vi "Connection Handler VI.vi"(9 "Additional Data":variant, 10 "connection ID":T1, 11 "TCP Server Refnum":refnum<class "JKI TCP Server.lvclass">) -> ()   [LabVIEW 2020]
uses:
  <vilib>/addons/_JKI.lib/_JKI_lib_TCP_Server.llb/TCP Server Connection Session ID Cluster.ctl
  <vilib>/addons/_JKI.lib/_JKI_lib_TCP_Server.llb/JKI TCP Server.lvclass
  bd168d05-2ccd-4f69-90c9-be1b4e621865.vi
  316abe05-dd11-44a4-98b3-32ea1594dc48.vi
  a7f8194b-54d4-448d-8a65-d0b66a8fd47c.vi
  8a9da1d4-9237-4126-a3a1-8a9d876b672d.vi
  eb58fbab-51b7-4bfd-aab6-475a21a34b28.vi
  <userlib>/_NEVSTOP/Communicable State Machine(CSM)/_Support/Common/Trim Single line Text.vi
  <userlib>/_NEVSTOP/Communicable State Machine(CSM)/AdvanceAPI/CSM - Make String Arguments Safe.vi
  <userlib>/_NEVSTOP/Communicable State Machine(CSM)/AdvanceAPI/CSM - Keywords.vi
  <userlib>/_NEVSTOP/Communicable State Machine(CSM)/addons/API-String-Arugments-Support/_Support/Data To API String Arguments.vi
  _support/Module/CSM-TCP-Router.lvlib
  <userlib>/_NEVSTOP/Communicable State Machine(CSM)/Communicable State Machine.lvlib
  <userlib>/_NEVSTOP/Communicable State Machine(CSM)/_csmHelper/API with lvcsm Support/CSM-Helper API with lvcsm Support.lvlib
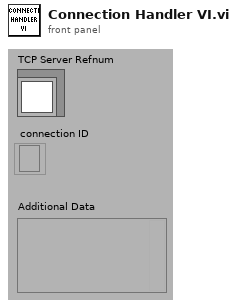
[diagram p1: front panel]
types:
  T1 = typedef "JKI TCP Server.lvclass/TCP Server Connection Session ID Cluster.ctl" = refnum<k5>
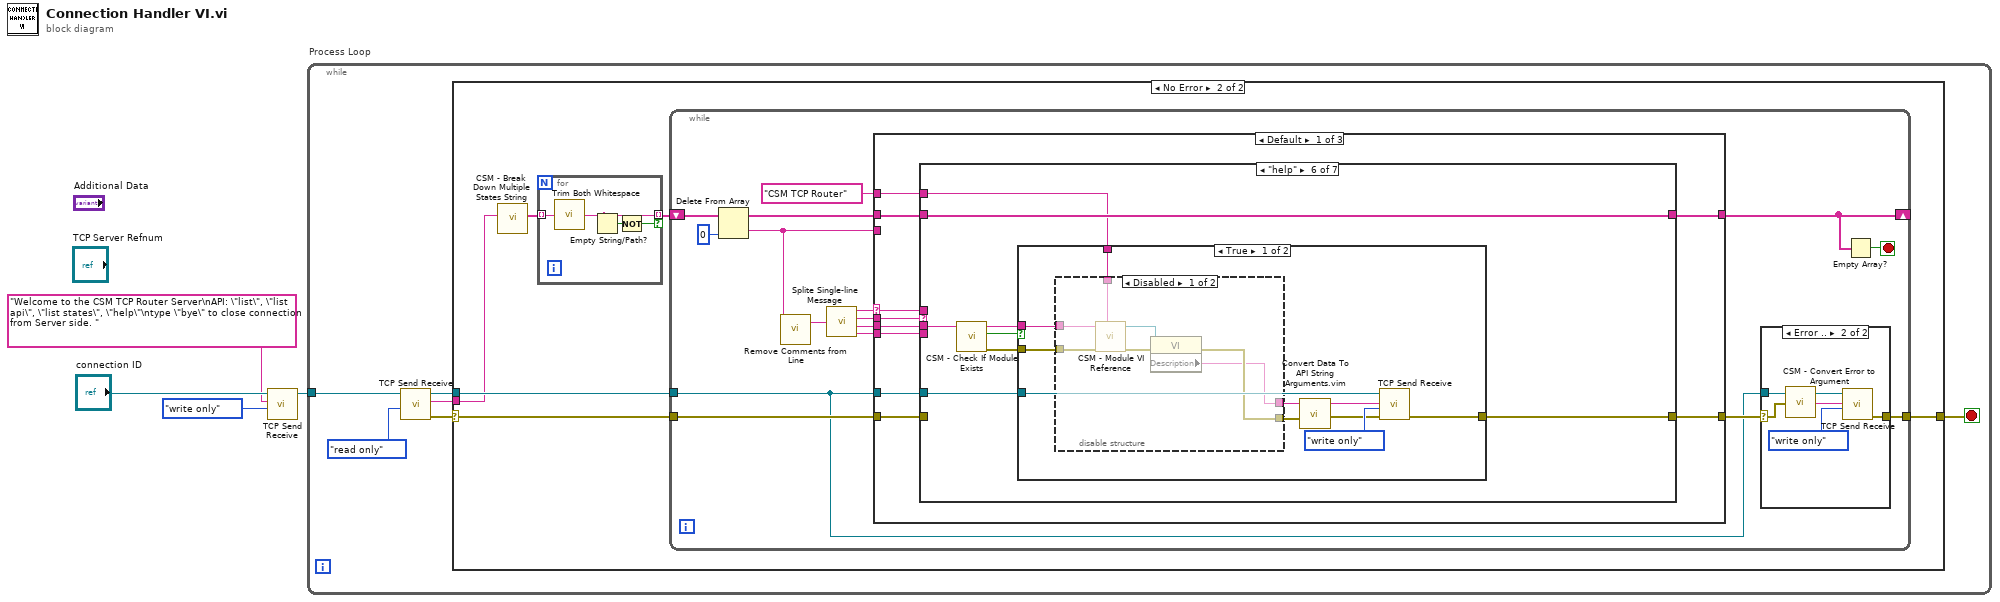
[diagram p0: block diagram]
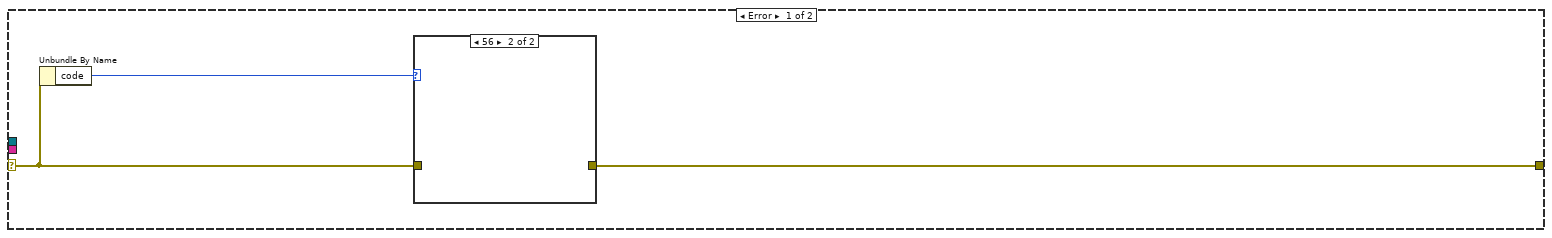
[diagram p2: hidden frame]
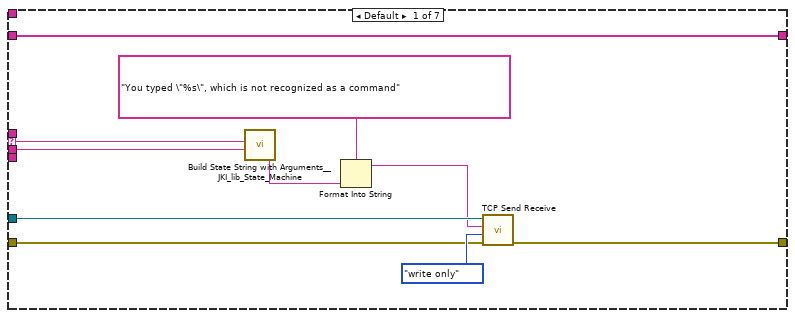
[diagram p5: hidden frame]
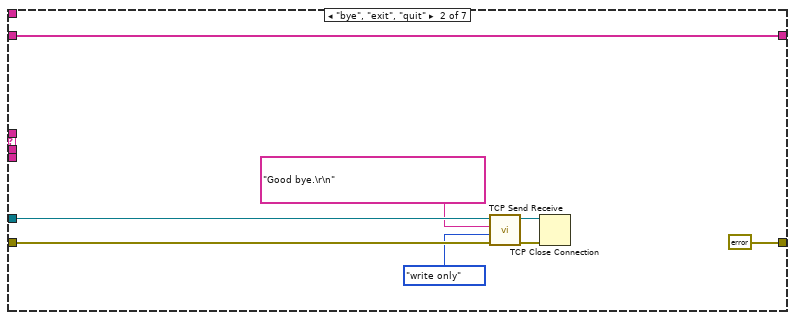
[diagram p6: hidden frame]
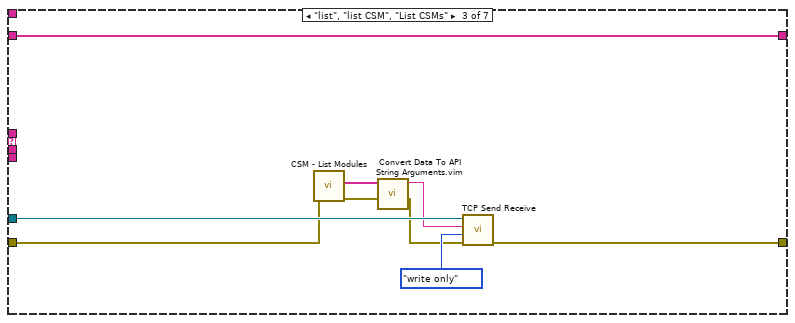
[diagram p7: hidden frame]
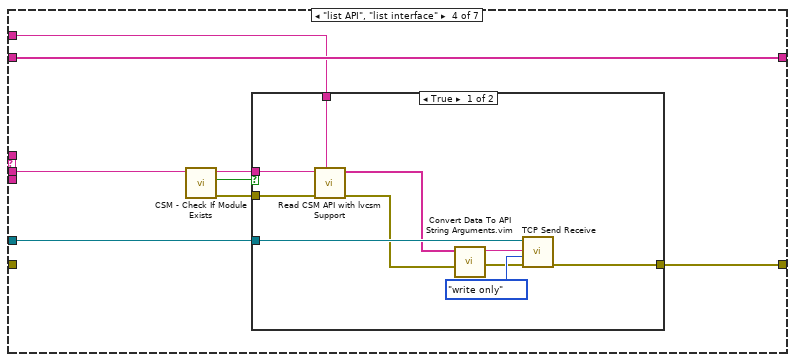
[diagram p8: hidden frame]
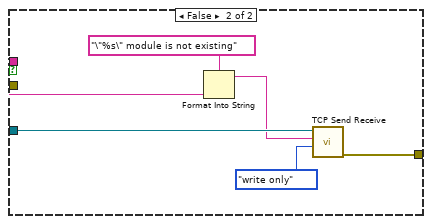
[diagram p9: hidden frame]
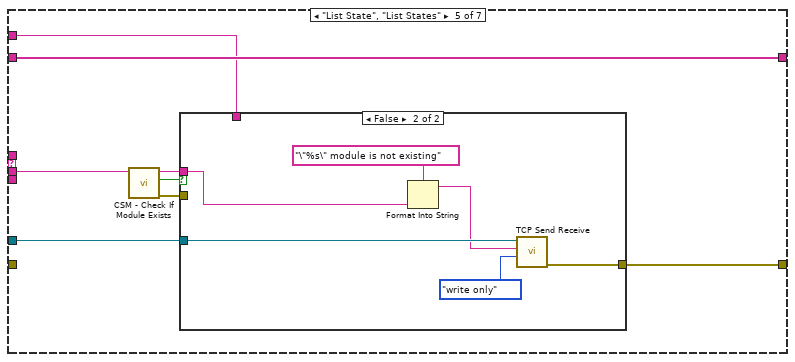
[diagram p10: hidden frame]
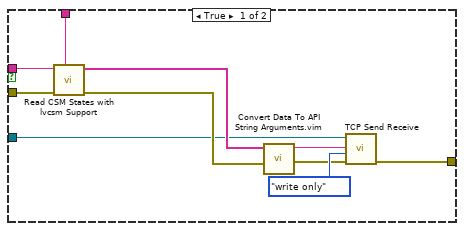
[diagram p11: hidden frame]
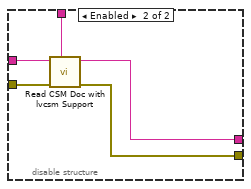
[diagram p12: hidden frame]
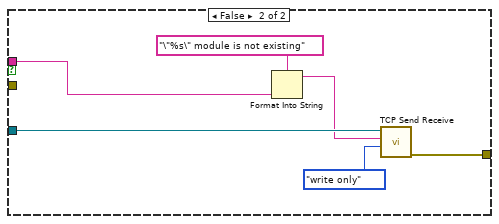
[diagram p13: hidden frame]
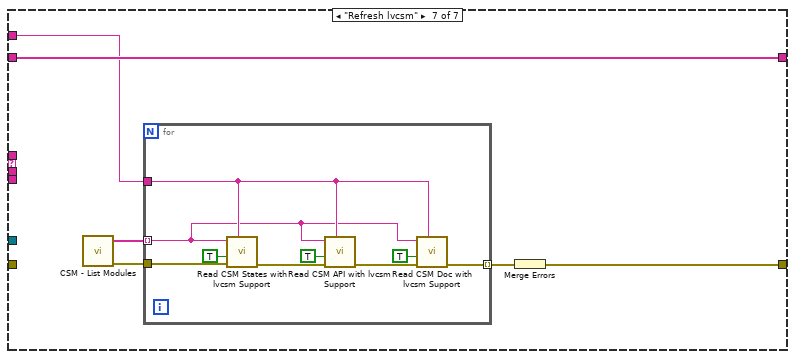
[diagram p14: hidden frame]
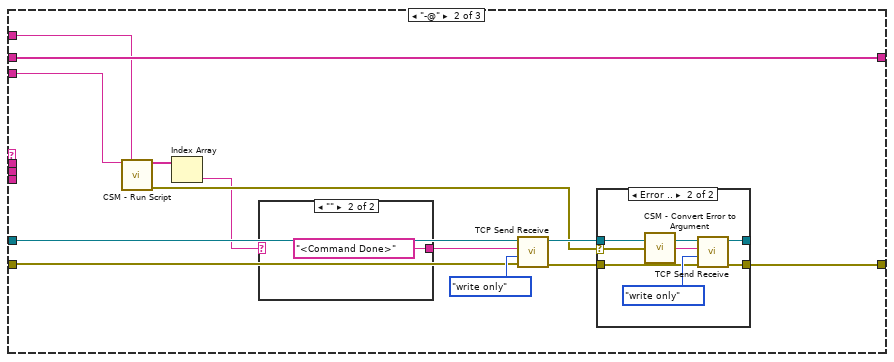
[diagram p15: hidden frame]
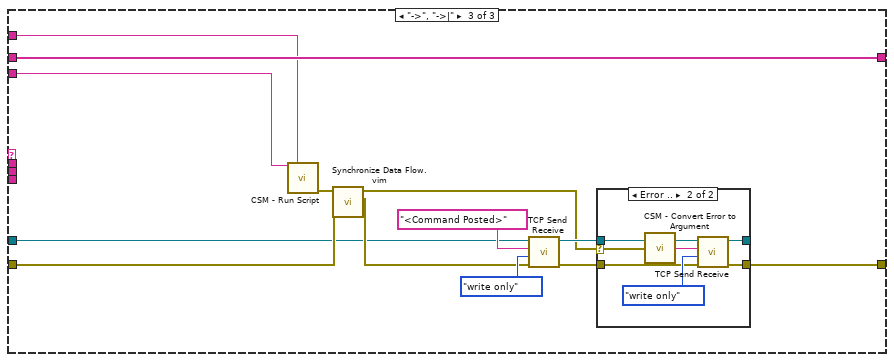
[diagram p18: hidden frame]
diagram:
  n1 = call "TCP Send Receive.vi"("access (read/write)"=enum16{"read/write", "read only", "write only"}."write only", "Data In"="Welcome to the CSM TCP Router Server\nAPI: \"list\", \"list api\", \"list states\", \"help\"\ntype \"bye\" to close connection from Server side. " ("data in"), "connection ID"="connection ID") -> ("connection ID Out"=w3:refnum<k5>)  [unwired: 6 in, 2 out]
  n2 = while "Process Loop" {
    tunnel: w3 -> [w9]
    stop <- w10 stop-if-true
    n3 = call "TCP Send Receive.vi"("access (read/write)"=enum16{"read/write", "read only", "write only"}."read only", "connection ID"=w9) -> ("error out"=w6:errorcluster, "Data Out"=w5:string, "connection ID Out"=w8:refnum<k5>)  [unwired: 7 in]
    n4 = case shown="No Error" w6 {
      selector: w6 -> [w12 w18]
      tunnel: w8 -> [_ w20]
      tunnel: w5 -> [_ w17]
      tunnel: [w11 w19] -> w10
      frame Error {
        n5 = Unbundle By Name(w12) -> ("code"=w13:i32)
        n6 = case shown="56" w13 {
          tunnel: w12 -> [w14 _]
          tunnel: [w14 _] -> w11
          frame 0, Default {
          }
          frame 56 {
          }
        }
      }
      frame No Error {
        n7 = call <userlib>:"CSM - Break Down Multiple States String.vi"("States"=w17) -> ("Multiple States"=w16:string[])  [unwired: 10 in]
        n8 = for {
          tunnel: w16 -> [w24] mode=indexing
          tunnel: [w23] -> w15 mode=indexing if=w21
          n9 = call <userlib>:"Trim Both Whitespace.vi"("string"=w24) -> ("trimmed string"=w23:string)  [unwired: 1 in]
          n10 = Empty String/Path?(string/path=w23) -> (empty?=w22:bool)
          n11 = Not(x=w22) -> (.not. x?=w21:bool)
        }
        n12 = while {
          tunnel: w20 -> [w27]
          tunnel: w18 -> [w40]
          tunnel: [w28] -> w19
          shift-right: [w30] -> _
          shift-left: w15 -> [w34]
          stop <- w31 stop-if-true
          n13 = Delete From Array(array=w34, index=0) -> (deleted portion=w26:string, array with subset deleted=w33:string[])  [unwired: 1 in]
          n14 = call <userlib>:"Remove Comments from Line.vi"("single-line text"=w26) -> ("single-line text without comments"=w39:string)  [unwired: 2 in]
          n15 = call <userlib>:"Splite Single-line Message.vi"("single-line text"=w39) -> ("operator"=w38:string, "state"=w37:string, "args"=w36:string, "source/target"=w35:string)  [unwired: 6 in]
          n16 = case shown="Default" w38 {
            selector: w38 -> [w50 _ _]
            tunnel: w27 -> [w56 w194 w207]
            tunnel: [w55 w191 w216] -> w29
            tunnel: w40 -> [w54 w187 w213]
            tunnel: w37 -> [w53 _ _]
            tunnel: w36 -> [w52 _ _]
            tunnel: w35 -> [w51 _ _]
            tunnel: [w49 w188 w214] -> w30
            tunnel: w33 -> [w48 w188 w214]
            tunnel: w26 -> [_ w186 w212]
            tunnel: "CSM TCP Router" ("Current Module(\"\" to generate a ID)") -> [w47 w185 w211]
            frame Default {
              n17 = case shown="\"help\"" w53 {
                selector: w53 -> [w63 _ _ _ _ _ _]
                tunnel: w56 -> [w66 w72 w83 w91 w115 w139 _]
                tunnel: [w65 errorcluster {"status"=TRUE, "code"=0, "source"=""} ("error out") w76 w90 w114 w138 w169] -> w55
                tunnel: w54 -> [w57 w73 w81 _ _ _ _]
                tunnel: w52 -> [w64 _ _ w86 w110 w134 _]
                tunnel: w51 -> [_ _ _ _ _ _ _]
                tunnel: w50 -> [_ _ _ _ _ _ _]
                tunnel: [w62 w69 w75 w89 w113 w137 w173] -> w49
                tunnel: w48 -> [w62 w69 w75 w89 w113 w137 w173]
                tunnel: w47 -> [_ _ _ w84 w108 w132 w168]
                frame Default {
                  n18 = call <vilib>:"Build State String with Arguments__JKI_lib_State_Machine.vi"("Arguments (\"\")"=w64, "State"=w63) -> ("State with Arguments"=w58:string)  [unwired: 4 in]
                  n19 = Format Into String(format string="You typed \"%s\", which is not recognized as a command", w58) -> (resulting string=w59:string)  [unwired: 2 in, 1 out]
                  n20 = call "TCP Send Receive.vi"("error in (no error)"=w57, "access (read/write)"=enum16{"read/write", "read only", "write only"}."write only", "Data In"=w59, "connection ID"=w66) -> ("error out"=w65:errorcluster)  [unwired: 5 in, 2 out]
                }
                frame "bye", "exit", "quit" {
                  n21 = call "TCP Send Receive.vi"("error in (no error)"=w73, "access (read/write)"=enum16{"read/write", "read only", "write only"}."write only", "Data In"="Good bye.\r\n" ("data in"), "connection ID"=w72) -> ("error out"=w68:errorcluster, "connection ID Out"=w67:refnum<k5>)  [unwired: 5 in, 1 out]
                  n22 = TCP Close Connection(connection ID=w67, error in (no error)=w68) -> ()  [unwired: 1 in, 2 out]
                }
                frame "list", "list CSM", "List CSMs" {
                  n23 = call <userlib>:"CSM - List Modules.vi"("Error in"=w81) -> ("Error out"=w79:errorcluster, "Module Names"=w80:string[])  [unwired: 9 in]
                  n24 = call "Convert Data To API String Arguments.vim"("error in (no error)"=w79, "data"=w80) -> ("error out"=w78:errorcluster, "String"=w77:string)  [unwired: 6 in]
                  n25 = call "TCP Send Receive.vi"("error in (no error)"=w78, "access (read/write)"=enum16{"read/write", "read only", "write only"}."write only", "Data In"=w77, "connection ID"=w83) -> ("error out"=w76:errorcluster)  [unwired: 5 in, 2 out]
                }
                frame "list API", "list interface" {
                  n26 = call <userlib>:"CSM - Check If Module Exists.vi"("CSM Name"=w86) -> ("Error out"=w88:errorcluster, "Exist?"=w85:bool, "CSM Name(dup)"=w87:string)  [unwired: 8 in]
                  n27 = case shown="True" w85 {
                    tunnel: w91 -> [w101 w107]
                    tunnel: [w100 w106] -> w90
                    tunnel: w88 -> [w96 _]
                    tunnel: w87 -> [w95 w102]
                    tunnel: w84 -> [w92 _]
                    frame True {
                      n28 = call <userlib>:"Read CSM API with lvcsm Support.vi"("Current Module(\"\" to generate a ID)"=w92, "error in (no error)"=w96, "CSM Name"=w95) -> ("Error out"=w94:errorcluster, "CSMAPI List"=w93:string[])  [unwired: 7 in]
                      n29 = call "Convert Data To API String Arguments.vim"("error in (no error)"=w94, "data"=w93) -> ("error out"=w98:errorcluster, "String"=w97:string)  [unwired: 6 in]
                      n30 = call "TCP Send Receive.vi"("error in (no error)"=w98, "access (read/write)"=enum16{"read/write", "read only", "write only"}."write only", "Data In"=w97, "connection ID"=w101) -> ("error out"=w100:errorcluster)  [unwired: 5 in, 2 out]
                    }
                    frame False {
                      n31 = Format Into String(format string="\"%s\" module is not existing", w102) -> (resulting string=w103:string)  [unwired: 2 in, 1 out]
                      n32 = call "TCP Send Receive.vi"("access (read/write)"=enum16{"read/write", "read only", "write only"}."write only", "Data In"=w103, "connection ID"=w107) -> ("error out"=w106:errorcluster)  [unwired: 6 in, 2 out]
                    }
                  }
                }
                frame "List State", "List States" {
                  n33 = call <userlib>:"CSM - Check If Module Exists.vi"("CSM Name"=w110) -> ("Error out"=w112:errorcluster, "Exist?"=w109:bool, "CSM Name(dup)"=w111:string)  [unwired: 8 in]
                  n34 = case shown="False" w109 {
                    tunnel: w115 -> [w117 w131]
                    tunnel: [w125 w130] -> w114
                    tunnel: w112 -> [w120 _]
                    tunnel: w111 -> [w119 w126]
                    tunnel: w108 -> [w116 _]
                    frame True {
                      n35 = call <userlib>:"Read CSM States with lvcsm Support.vi"("Current Module(\"\" to generate a ID)"=w116, "error in (no error)"=w120, "CSM Name"=w119) -> ("Error out"=w118:errorcluster, "CSMAPI List"=w121:string[])  [unwired: 7 in]
                      n36 = call "Convert Data To API String Arguments.vim"("error in (no error)"=w118, "data"=w121) -> ("error out"=w123:errorcluster, "String"=w122:string)  [unwired: 6 in]
                      n37 = call "TCP Send Receive.vi"("error in (no error)"=w123, "access (read/write)"=enum16{"read/write", "read only", "write only"}."write only", "Data In"=w122, "connection ID"=w117) -> ("error out"=w125:errorcluster)  [unwired: 5 in, 2 out]
                    }
                    frame False {
                      n38 = Format Into String(format string="\"%s\" module is not existing", w126) -> (resulting string=w127:string)  [unwired: 2 in, 1 out]
                      n39 = call "TCP Send Receive.vi"("access (read/write)"=enum16{"read/write", "read only", "write only"}."write only", "Data In"=w127, "connection ID"=w131) -> ("error out"=w130:errorcluster)  [unwired: 6 in, 2 out]
                    }
                  }
                }
                frame "help" {
                  n40 = call <userlib>:"CSM - Check If Module Exists.vi"("CSM Name"=w134) -> ("Error out"=w136:errorcluster, "Exist?"=w133:bool, "CSM Name(dup)"=w135:string)  [unwired: 8 in]
                  n41 = case shown="True" w133 {
                    tunnel: w139 -> [w143 w167]
                    tunnel: [w149 w166] -> w138
                    tunnel: w136 -> [w145 _]
                    tunnel: w135 -> [w144 w162]
                    tunnel: w132 -> [w140 _]
                    frame True {
                      n42 = disable-structure shown="Disabled" {
                        disable-tunnel: w145 -> [w156 w161]
                        disable-tunnel: w144 -> [w155 w160]
                        disable-tunnel: [w153 w158] -> w142
                        disable-tunnel: [w151 w157] -> w141
                        disable-tunnel: w140 -> [w150 w159]
                        frame Disabled {
                          n43 = call <userlib>:"CSM - Module VI Reference.vi"("Current Module(\"\" to generate a ID)"=w150, "error in (no error)"=w156, "CSM Name"=w155) -> ("error out"=w154:errorcluster, "CSM Module VIRef"=w152:refnum<vi>)  [unwired: 7 in]
                          n44 = property class="VI"(reference=w152, error in=w154) -> (error out=w153:errorcluster, "Description"=w151:string)  [unwired: 1 out]
                        }
                        frame Enabled {
                          n45 = call "Read CSM Doc with lvcsm Support.vi"("Current Module(\"\" to generate a ID)"=w159, "error in (no error)"=w161, "CSM Name"=w160) -> ("Error out"=w158:errorcluster, "CSM Doc"=w157:string)  [unwired: 7 in]
                        }
                      }
                      n46 = call "Convert Data To API String Arguments.vim"("error in (no error)"=w142, "data"=w141) -> ("error out"=w147:errorcluster, "String"=w146:string)  [unwired: 6 in]
                      n47 = call "TCP Send Receive.vi"("error in (no error)"=w147, "access (read/write)"=enum16{"read/write", "read only", "write only"}."write only", "Data In"=w146, "connection ID"=w143) -> ("error out"=w149:errorcluster)  [unwired: 5 in, 2 out]
                    }
                    frame False {
                      n48 = Format Into String(format string="\"%s\" module is not existing", w162) -> (resulting string=w163:string)  [unwired: 2 in, 1 out]
                      n49 = call "TCP Send Receive.vi"("access (read/write)"=enum16{"read/write", "read only", "write only"}."write only", "Data In"=w163, "connection ID"=w167) -> ("error out"=w166:errorcluster)  [unwired: 6 in, 2 out]
                    }
                  }
                }
                frame "Refresh lvcsm" {
                  n50 = call <userlib>:"CSM - List Modules.vi"() -> ("Error out"=w172:errorcluster, "Module Names"=w171:string[])  [unwired: 10 in]
                  n51 = for {
                    tunnel: w172 -> [w182]
                    tunnel: w171 -> [w175] mode=indexing
                    tunnel: [w177] -> w170 mode=indexing
                    tunnel: w168 -> [w176]
                    n52 = call <userlib>:"Read CSM States with lvcsm Support.vi"("Current Module(\"\" to generate a ID)"=w176, "error in (no error)"=w182, "Force?(F)"=TRUE, "CSM Name"=w175) -> ("Error out"=w181:errorcluster)  [unwired: 6 in, 1 out]
                    n53 = call <userlib>:"Read CSM API with lvcsm Support.vi"("Current Module(\"\" to generate a ID)"=w176, "error in (no error)"=w181, "Force?(F)"=TRUE, "CSM Name"=w175) -> ("Error out"=w178:errorcluster)  [unwired: 6 in, 1 out]
                    n54 = call "Read CSM Doc with lvcsm Support.vi"("Current Module(\"\" to generate a ID)"=w176, "error in (no error)"=w178, "Force?(F)"=TRUE, "CSM Name"=w175) -> ("Error out"=w177:errorcluster)  [unwired: 6 in, 1 out]
                  }
                  n55 = Merge Errors(w170) -> (w169:errorcluster)
                }
              }
            }
            frame "-@" {
              n56 = call <userlib>:"CSM - Run Script.vi"("CSM Scripts"=w186, "Current Module(\"\" to generate a ID)"=w185) -> ("Response"=w184:string[], "error out"=w190:errorcluster)  [unwired: 11 in, 1 out]
              n57 = Index Array(array=w184) -> (element=w183:string)  [unwired: 1 in]
              n58 = case shown="\"\"" w183 {
                selector: w183 -> [w196 _]
                tunnel: [w196 "<Command Done>"] -> w189
                frame Default {
                }
                frame "" {
                }
              }
              n59 = call "TCP Send Receive.vi"("error in (no error)"=w187, "access (read/write)"=enum16{"read/write", "read only", "write only"}."write only", "Data In"=w189, "connection ID"=w194) -> ("error out"=w193:errorcluster, "connection ID Out"=w192:refnum<k5>)  [unwired: 5 in, 1 out]
              n60 = case shown="Error .." w190 {
                selector: w190 -> [_ w202]
                tunnel: w193 -> [w199 w205]
                tunnel: w192 -> [w198 w204]
                tunnel: [w199 w203] -> w191
                tunnel: [w198 w200] -> _
                frame No Error {
                }
                frame Error {
                  n61 = call <userlib>:"CSM - Convert Error to Argument.vi"("error"=w202) -> ("Argument"=w201:string)  [unwired: 4 in]
                  n62 = call "TCP Send Receive.vi"("error in (no error)"=w205, "access (read/write)"=enum16{"read/write", "read only", "write only"}."write only", "Data In"=w201, "connection ID"=w204) -> ("error out"=w203:errorcluster, "connection ID Out"=w200:refnum<k5>)  [unwired: 5 in, 1 out]
                }
              }
            }
            frame "->", "->|" {
              n63 = call <userlib>:"CSM - Run Script.vi"("CSM Scripts"=w212, "Current Module(\"\" to generate a ID)"=w211) -> ("error out"=w209:errorcluster)  [unwired: 11 in, 2 out]
              n64 = call "Synchronize Data Flow.vim"("input 2"=w213, "input 1"=w209) -> ("output 2"=w210:errorcluster, "output 1"=w208:errorcluster)  [unwired: 2 in, 2 out]
              n65 = call "TCP Send Receive.vi"("error in (no error)"=w210, "access (read/write)"=enum16{"read/write", "read only", "write only"}."write only", "Data In"="<Command Posted>", "connection ID"=w207) -> ("error out"=w218:errorcluster, "connection ID Out"=w217:refnum<k5>)  [unwired: 5 in, 1 out]
              n66 = case shown="Error .." w208 {
                selector: w208 -> [_ w224]
                tunnel: w218 -> [w221 w227]
                tunnel: w217 -> [w220 w226]
                tunnel: [w221 w225] -> w216
                tunnel: [w220 w222] -> _
                frame No Error {
                }
                frame Error {
                  n67 = call <userlib>:"CSM - Convert Error to Argument.vi"("error"=w224) -> ("Argument"=w223:string)  [unwired: 4 in]
                  n68 = call "TCP Send Receive.vi"("error in (no error)"=w227, "access (read/write)"=enum16{"read/write", "read only", "write only"}."write only", "Data In"=w223, "connection ID"=w226) -> ("error out"=w225:errorcluster, "connection ID Out"=w222:refnum<k5>)  [unwired: 5 in, 1 out]
                }
              }
            }
          }
          n69 = case shown="Error .." w29 {
            selector: w29 -> [w41 w42]
            tunnel: w27 -> [_ w45]
            tunnel: [w41 w44] -> w28
            frame No Error {
            }
            frame Error {
              n70 = call <userlib>:"CSM - Convert Error to Argument.vi"("error"=w42) -> ("Argument"=w43:string)  [unwired: 4 in]
              n71 = call "TCP Send Receive.vi"("access (read/write)"=enum16{"read/write", "read only", "write only"}."write only", "Data In"=w43, "connection ID"=w45) -> ("error out"=w44:errorcluster)  [unwired: 6 in, 2 out]
            }
          }
          n72 = Empty Array?(array=w30) -> (empty?=w31:bool)
        }
      }
    }
  }
